vi "niRFUtil RFHS Channelizer GetFilterType.vi"(0 "fs":dbl=1.0, 2 "Benchmark Task":T1, 5 "Channel Specification":T3={"fc"=0.0, "fs"=1.0, "passBW"=0.0, "stopBW"=0.0, "Rejection (dB)"=0.0, "Flags"=0, "Reserved"=0} {"Flags" items=["None"=0, "Force Fractional"=1, "Use Multistage"=2, "Use Pretrigger Data "=256, "Frequency Shift Only"=4]; "fs" format="%#_8p"; "fc" format="%#_6p"; "stopBW" format="%#_6p"; "passBW" format="%#_6p"}) -> (4 "Fractional":bool, 6 "Filter Spec":T2 {"Spec"."Flags" items=["None"=0, "Force Fractional"=1, "Use Multistage"=2, "Use Pretrigger Data "=256, "Frequency Shift Only"=4]; "Spec"."fs" format="%#_8p"; "Spec"."fc" format="%#_6p"; "Spec"."stopBW" format="%#_6p"; "Spec"."passBW" format="%#_6p"}, 8 "Upsample":i32, 10 "Downsample":dbl)   [LabVIEW 2015, in "niRFUtil.lvlib"]
uses:
  niRFUtil.lvlib
  Includes/niRFUtil RFHS Channelizer ChannelSpecificationBase.ctl
  Includes/niRFUtil RFHS Channelizer ChannelFlags.ctl
  Includes/niRFUtil RFHS Channelizer FilterSpecification.ctl
  Utilities/Benchmark/niRFUtil RFHS Benchmark Task.ctl
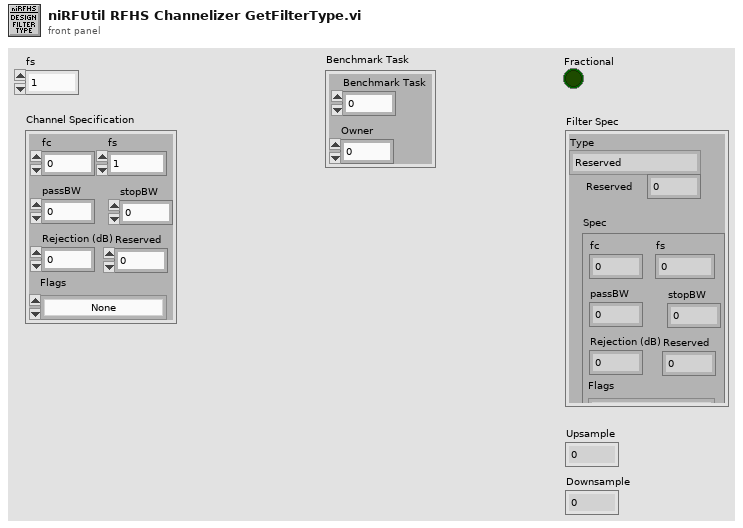
[diagram p1: front panel]
types:
  T1 = typedef "niRFUtil.lvlib/niRFUtil RFHS Benchmark Task.ctl" = cluster{"Benchmark Task":u64, "Owner":u32}
  T2 = typedef "niRFUtil.lvlib/niRFUtil RFHS Channelizer FilterSpecification.ctl" = cluster{"Type":enum32{"Reserved", "Rational", "Fine Tune", "Fractional", "Rational (user)", "Reserved 2", "Fractional (user)", "FFT Resampler"}, "Reserved":i32, "Spec":T3}
  T3 = typedef "niRFUtil.lvlib/niRFUtil RFHS Channelizer ChannelSpecificationBase.ctl" = cluster{"fc":dbl, "fs":dbl, "passBW":dbl, "stopBW":dbl, "Rejection (dB)":dbl, "Flags":T4, "Reserved":i32}
  T4 = typedef "niRFUtil.lvlib/niRFUtil RFHS Channelizer ChannelFlags.ctl" = u32
  T5 = enum16{"Reserved", "Rational", "Fine Tune", "Fractional"}
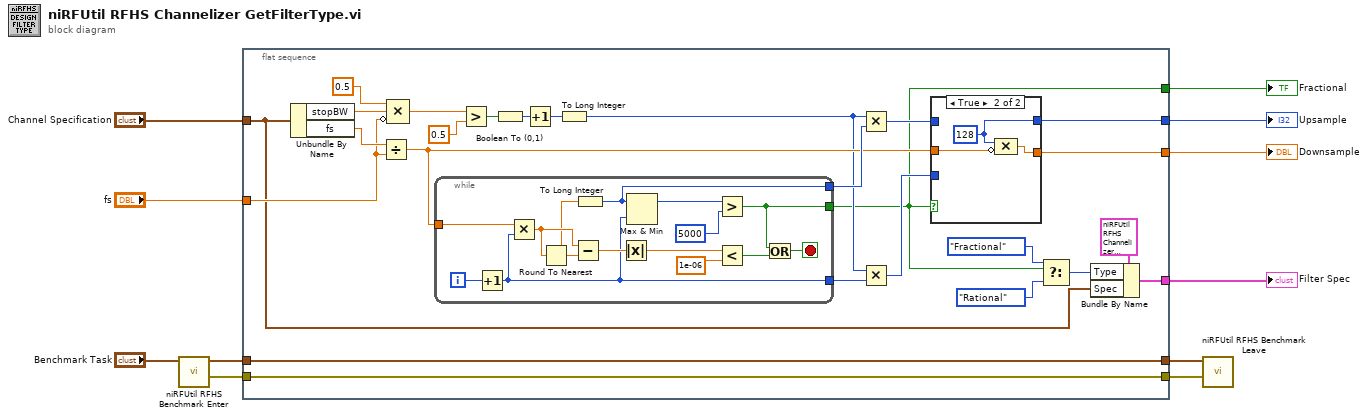
[diagram p0: block diagram]
diagram:
  n1 = call "niRFUtil RFHS Benchmark Enter.vi"("Benchmark Task (Parent)"="Benchmark Task") -> ("error out"=w2:errorcluster, "Benchmark Task (Self)"=w4:T1)  [unwired: 9 in]
  n2 = flat-sequence {
    tunnel: "fs" -> [w34]
    tunnel: [w32] -> w10
    tunnel: [w30] -> w9
    tunnel: "Channel Specification" -> [w27]
    tunnel: [w24] -> w7
    tunnel: [w13] -> w6
    tunnel: w4 -> [w18]
    tunnel: [w18] -> w3
    tunnel: w2 -> [w17]
    tunnel: [w17] -> w1
    frame #0 {
      n3 = Unbundle By Name(w27) -> ("stopBW"=w35:dbl, "fs"=w37:dbl)
      n4 = Divide(x=w37, y=w34) -> (x/y=w29:dbl)
      n5 = Compound Arithmetic op=MULTIPLY(0.5 ("value"), w35, invert w34) -> (w23:dbl)
      n6 = while {
        tunnel: w29 -> [w56]
        tunnel: [w48] -> w15
        tunnel: [w49] -> w36
        tunnel: [w44] -> w13
        i -> [w55]
        stop <- w45 stop-if-true
        n7 = Increment(x=w55) -> (x+1=w48:i32)
        n8 = Multiply(x=w56, y=w48) -> (x*y=w54:dbl)
        n9 = Round To Nearest(number=w54) -> (nearest integer value=w50:dbl)
        n10 = Subtract(x=w54, y=w50) -> (x-y=w51:dbl)
        n11 = To Long Integer(number=w50) -> (32bit integer=w49:i32)
        n12 = Absolute Value(x=w51) -> (abs(x)=w53:dbl)
        n13 = Max & Min(x=w49, y=w48) -> (max(x,y)=w47:i32)  [unwired: 1 out]
        n14 = Greater?(x=w47, y=5000) -> (0:w44:bool)
        n15 = Less?(x=w53, y=1e-06) -> (x < y?=w43:bool)
        n16 = Or(x=w44, y=w43) -> (x .or. y?=w45:bool)
      }
      n17 = Greater?(x=w23, y=0.5) -> (0:w21:bool)
      n18 = Boolean To (0,1)(Boolean=w21) -> (0, 1=w20:i16)
      n19 = Increment(x=w20) -> (x+1=w19:i16)
      n20 = To Long Integer(number=w19) -> (32bit integer=w14:i32)
      n21 = Multiply(x=w14, y=w36) -> (x*y=w31:i32)
      n22 = Multiply(x=w14, y=w15) -> (x*y=w33:i32)
      n23 = case shown="True" w13 {
        tunnel: w33 -> [w38 _]
        tunnel: [w38 w41] -> w32
        tunnel: w31 -> [w39 _]
        tunnel: [w39 w40] -> w30
        tunnel: w29 -> [_ w42]
        frame False {
        }
        frame True {
          w40 = 128
          n24 = Compound Arithmetic op=MULTIPLY(w40, invert w42) -> (w41:dbl)
        }
      }
      n25 = Select(t=T5."Fractional" ("Type"), s=w13, f=T5."Rational" ("Type")) -> (s? t:f=w12:T5)
      n26 = Bundle By Name(cluster=T2 {"Type"=enum."Reserved", "Reserved"=0, "Spec"={"fc"=0.0, "fs"=0.0, "passBW"=0.0, "stopBW"=0.0, "Rejection (dB)"=0.0, "Flags"=0, "Reserved"=0}} ("Filter Spec"), "Type"=w12, "Spec"=w27) -> (w24:T2)
    }
  }
  n27 = call "niRFUtil RFHS Benchmark Leave.vi"("error in (no error)"=w1, "Benchmark Task Self"=w3) -> ()  [unwired: 8 in, 2 out]
  "Fractional" <- w6
  "Downsample" <- w10
  "Upsample" <- w9
  "Filter Spec" <- w7
